vi "vis_com_RW.vi"(6 "SerialSetting":T1={"Baud Rate"=115200, "Data Bits"=8, "Parity"=0, "Stop Bits"=10} {"Stop Bits" items=["1.0"=10, "1.5"=15, "2.0"=20]; "Parity" items=["None", "Odd", "Even", "Mark", "Space"]}, 7 "Funciton":T2, 8 "error in (no error)":errorcluster, 9 "TermChar":string="\n", 10 "CMD String":string, 11 "VISA resource in":refnum<visa-resource-name>) -> (0 "error out":errorcluster, 2 "Result":string, 3 "VISA resource out":refnum<visa-resource-name>)   [LabVIEW 2020, in "GPP.lvlib"]
uses:
  GPP.lvlib
  VISA_COMMON.ctl
  Global.vi
panel:
  out "trimmed string":string
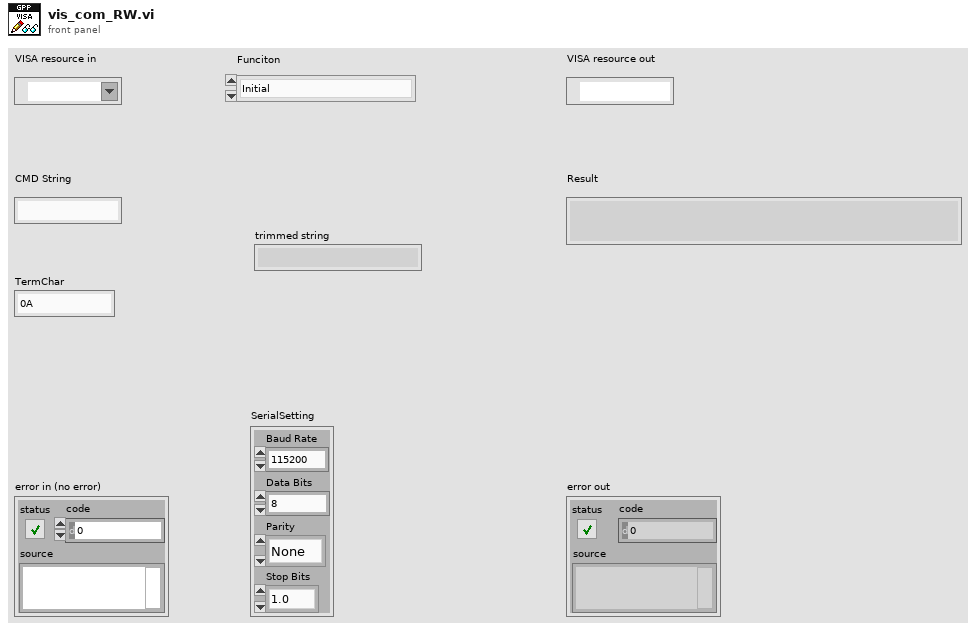
[diagram p1: front panel]
types:
  T1 = cluster{"Baud Rate":u32, "Data Bits":u16, "Parity":u16, "Stop Bits":u16}
  T2 = typedef "GPP.lvlib/VISA_COMMON.ctl" = enum16{"Initial", "Write CMD", "Read Result", "Read History", "Close"}
  T3 = enum16{"open", "replace", "create", "open or create", "replace or create", "replace or create with confirmation"}
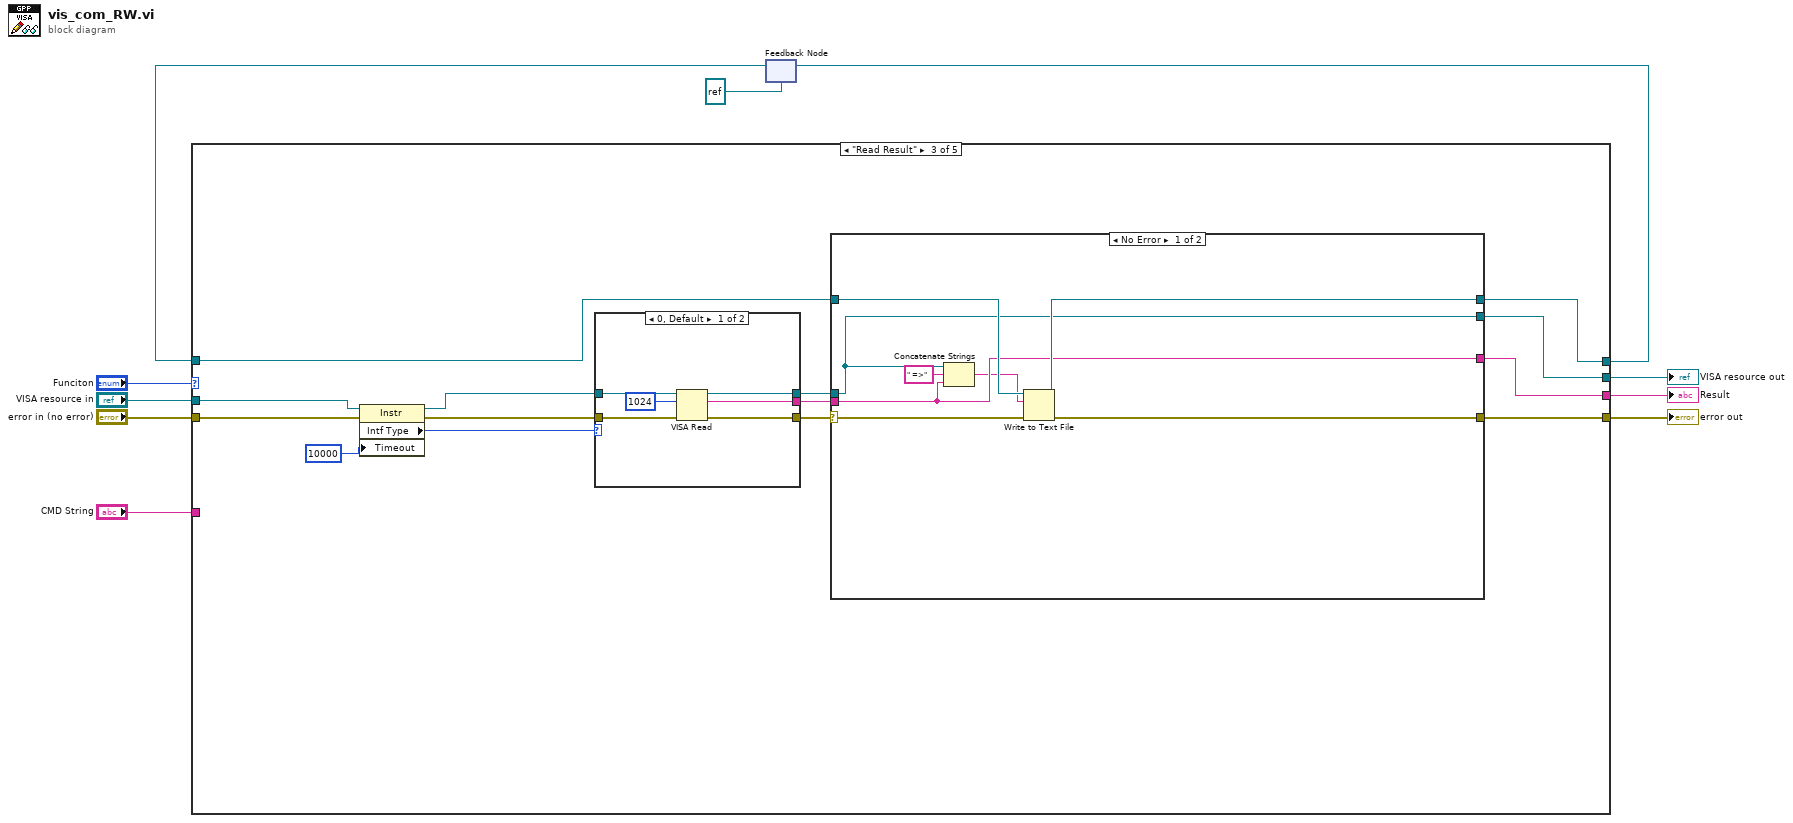
[diagram p0: block diagram]
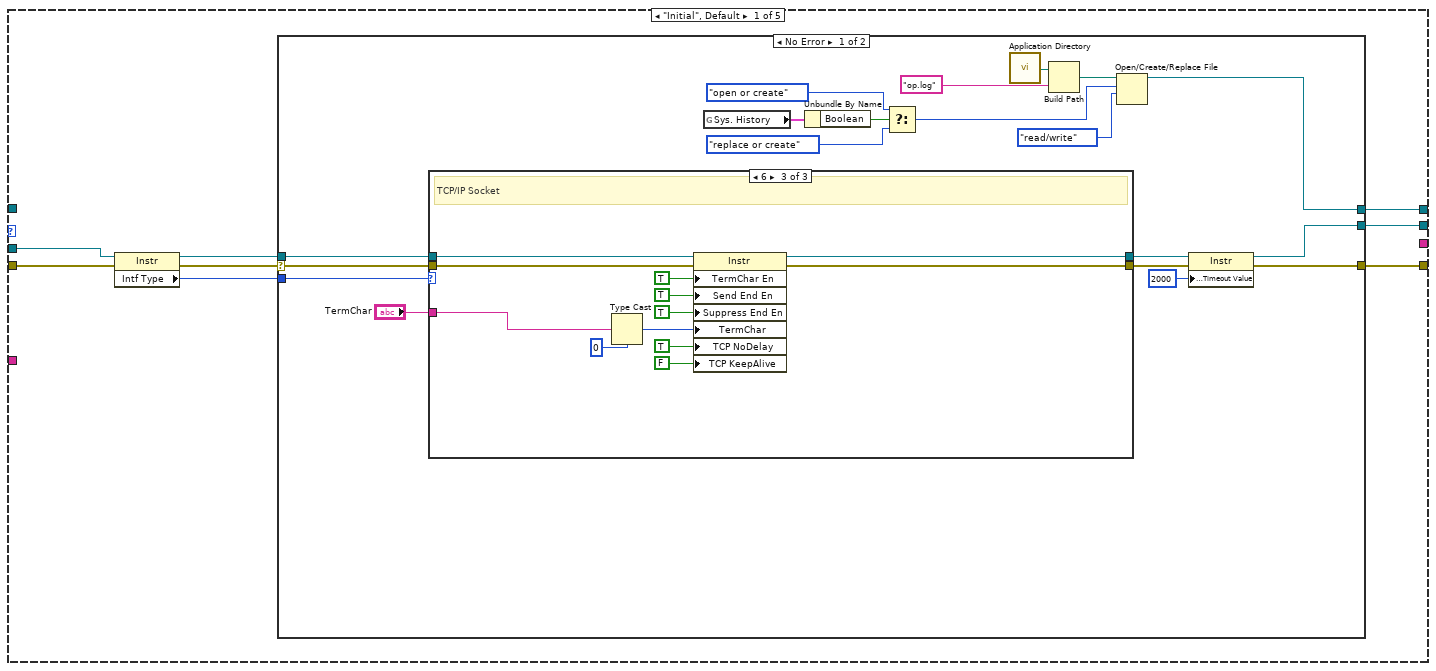
[diagram p2: hidden frame]
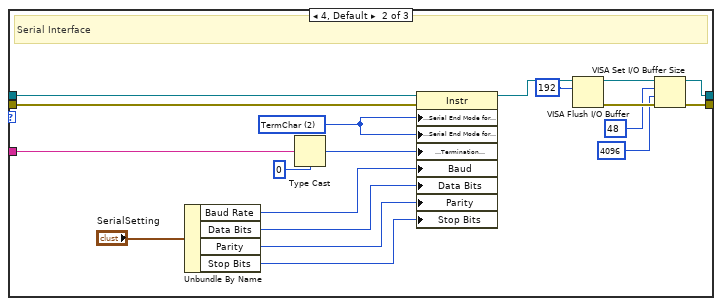
[diagram p4: hidden frame]
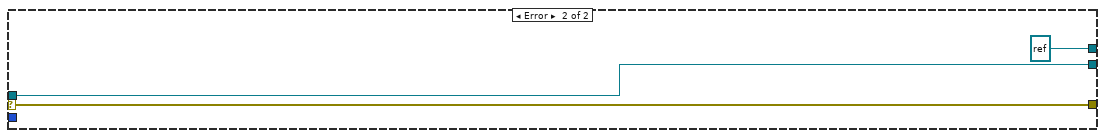
[diagram p5: hidden frame]
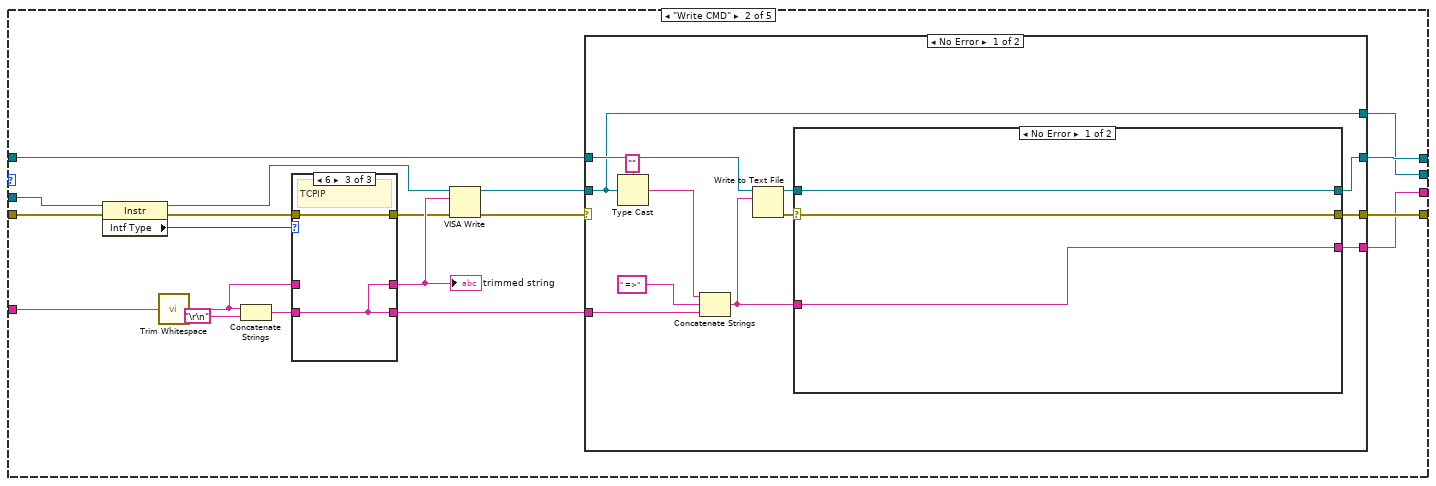
[diagram p6: hidden frame]
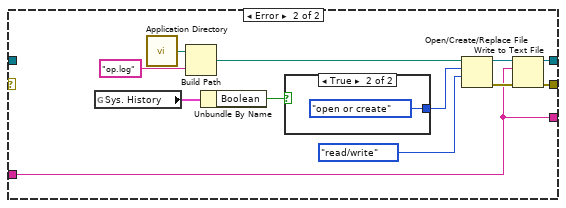
[diagram p9: hidden frame]
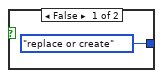
[diagram p10: hidden frame]
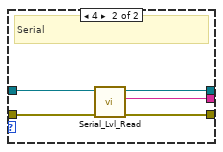
[diagram p12: hidden frame]
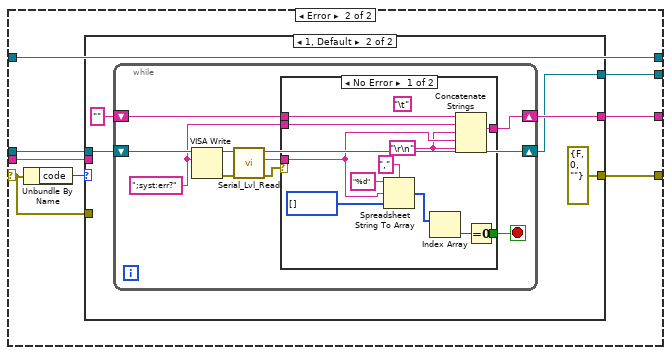
[diagram p13: hidden frame]
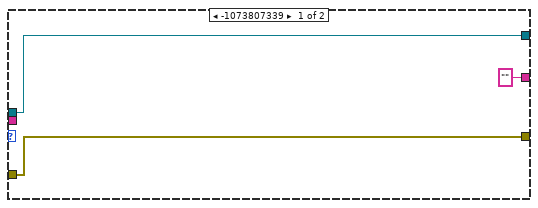
[diagram p14: hidden frame]
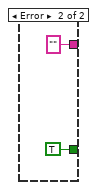
[diagram p15: hidden frame]
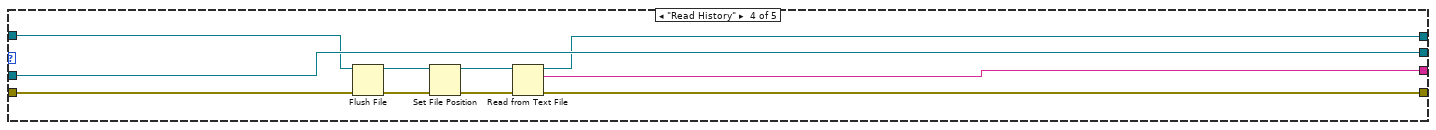
[diagram p16: hidden frame]
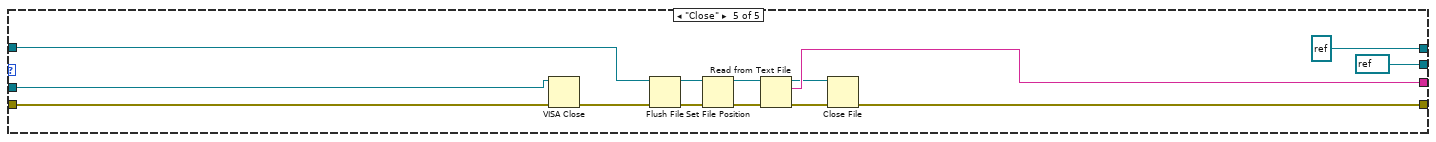
[diagram p17: hidden frame]
diagram:
  n1 = feedback #1(refnum<file> refnum ("refnum out")) -> (w4:refnum<file>)
  n2 = case shown="\"Read Result\"" "Funciton" {
    tunnel: "VISA resource in" -> [w17 w85 w145 w211 w227]
    tunnel: "CMD String" -> [_ w83 _ _ _]
    tunnel: "error in (no error)" -> [w13 w84 w134 w204 w226]
    tunnel: [w12 w91 w143 w212 w221] -> w7
    tunnel: [_ w88 w142 w213 w225] -> w6
    tunnel: [w18 w90 w139 w205 refnum<file> refnum ("refnum out")] -> w3
    tunnel: w4 -> [_ w92 w141 w210 w217]
    tunnel: [w14 w86 w135 w211 refnum<visa-resource-name> refnum ("VISA resource out")] -> w1
    frame "Initial", Default {
      n3 = property class="Instr"(reference=w17, error in=w13) -> (reference out=w15:refnum<visa-resource-name>, error out=w11:errorcluster, "Intf Type"=w16:u16)
      n4 = case shown="No Error" w11 {
        selector: w11 -> [w22 w72]
        tunnel: [w33 refnum<file> refnum ("refnum out")] -> w18
        tunnel: w16 -> [w24 _]
        tunnel: w15 -> [w23 w73]
        tunnel: [w31 w73] -> w14
        tunnel: [w30 w72] -> w12
        frame No Error {
          n5 = case shown="6" w24 {
            tunnel: [w38 w55 w68] -> w21
            tunnel: [w39 w53 w67] -> w20
            tunnel: w23 -> [w38 w57 w70]
            tunnel: w22 -> [w39 w58 w69]
            tunnel: "TermChar" -> [_ w46 w59]
            frame 1 {
              # "GPIB and USB Interface"
            }
            frame 4, Default {
              w47 = u16 2 items=["None", "LastBit", "TermChar"] ("Serial Settings:Serial End Mode for Reads")
              # "Serial Interface"
              n6 = Unbundle By Name("SerialSetting") -> ("Baud Rate"=w44:u32, "Data Bits"=w43:u16, "Parity"=w42:u16, "Stop Bits"=w41:u16)
              n7 = Type Cast(type=u8 0, x=w46) -> (*(type *) &x=w40:u8)
              n8 = property class="Instr"(reference=w57, error in=w58, "Serial Settings:Serial End Mode for Reads"=w47, "Serial Settings:Serial End Mode for Writes"=w47, "Message Based Settings:Termination Character"=w40, "Baud"=w44, "Data Bits"=w43, "Parity"=w42, "Stop Bits"=w41) -> (reference out=w52:refnum<visa-resource-name>)  [unwired: 1 out]
              n9 = VISA Flush I/O Buffer(VISA resource name=w52, mask (16)=u16 192) -> (VISA resource name out=w56:refnum<visa-resource-name>, error out=w54:errorcluster)  [unwired: 1 in]
              n10 = VISA Set I/O Buffer Size(VISA resource name=w56, mask (16)=u16 48, size (4096)=u32 4096 ("size (0)"), error in (no error)=w54) -> (VISA resource name out=w55:refnum<visa-resource-name>, error out=w53:errorcluster)
            }
            frame 6 {
              # "TCP/IP Socket"
              n11 = Type Cast(type=u8 0, x=w59) -> (*(type *) &x=w65:u8)
              n12 = property class="Instr"(reference=w70, error in=w69, "TermChar En"=TRUE ("Message Based Settings:Termination Character Enable"), "Send End En"=TRUE ("Message Based Settings:Send End Enable"), "Suppress End En"=TRUE ("Message Based Settings:Suppress End Enable"), "TermChar"=w65, "TCP NoDelay"=TRUE ("TCP/IP Settings:No Packet Delay"), "TCP KeepAlive"=FALSE ("TCP/IP Settings:Keep-Alive Packets")) -> (reference out=w68:refnum<visa-resource-name>, error out=w67:errorcluster)
            }
          }
          n13 = global read "Global.vi" "Sys. History"() -> (w29:cluster{"Boolean":bool})
          n14 = Unbundle By Name(w29) -> ("Boolean"=w28:bool)
          n15 = Select(t=T3."open or create", s=w28, f=T3."replace or create" ("operation (0:open)")) -> (s? t:f=w27:T3)
          n16 = call <vilib>:"Application Directory.vi"() -> ("Application Directory"=w36:path)
          n17 = Build Path(base path=w36, name or relative path="op.log") -> (appended path=w37:path)
          n18 = Open/Create/Replace File(file path (use dialog)=w37, operation (0:open)=w27, access (0:read/write)=enum16{"read/write", "read-only", "write-only"}."read/write") -> (refnum out=w33:refnum<file>)  [unwired: 3 in, 2 out]
          n19 = property class="Instr"(reference=w21, error in=w20, "General Settings:Timeout Value"=u32 2000) -> (reference out=w31:refnum<visa-resource-name>, error out=w30:errorcluster)
        }
        frame Error {
        }
      }
    }
    frame "Write CMD" {
      n20 = property class="Instr"(reference=w85, error in=w84) -> (reference out=w75:refnum<visa-resource-name>, error out=w77:errorcluster, "Intf Type"=w74:u16)
      n21 = call <vilib>:"Trim Whitespace.vi"("string"=w83) -> ("trimmed string"=w79:string)  [unwired: 1 in]
      n22 = Concatenate Strings(w79, "\r\n") -> (w78:string)
      n23 = case shown="6" w74 {
        tunnel: w79 -> [w93 w97 _]
        tunnel: [w93 w96 w99] -> w81
        tunnel: [w93 w97 w99] -> w82
        tunnel: w78 -> [_ w96 w99]
        tunnel: w77 -> [w94 w95 w98]
        tunnel: [w94 w95 w98] -> w76
        frame 0, Default {
        }
        frame 4 {
          # "Serial"
        }
        frame 6 {
          # "TCPIP"
        }
      }
      "trimmed string" <- w82
      n24 = VISA Write(VISA resource name=w75, write buffer=w82, error in (no error)=w76) -> (VISA resource name out=w89:refnum<visa-resource-name>, error out=w87:errorcluster)  [unwired: 1 out]
      n25 = case shown="No Error" w87 {
        selector: w87 -> [_ w130]
        tunnel: w92 -> [w111 w131]
        tunnel: [w109 w130] -> w91
        tunnel: [w108 w131] -> w90
        tunnel: w81 -> [w106 _]
        tunnel: w89 -> [w101 w129]
        tunnel: [w105 _] -> w88
        tunnel: [w101 w129] -> w86
        frame No Error {
          n26 = Type Cast(type="" ("string"), x=w101) -> (*(type *) &x=w100:string)
          n27 = Concatenate Strings(w100, " =>" ("string"), w106) -> (w103:string)
          n28 = Write to Text File(file (use dialog)=w111, text=w103) -> (refnum out=w107:refnum<file>, error out=w110:errorcluster)  [unwired: 2 in, 1 out]
          n29 = case shown="No Error" w110 {
            selector: w110 -> [w114 _]
            tunnel: [w114 w122] -> w109
            tunnel: [w113 w120] -> w108
            tunnel: w107 -> [w113 _]
            tunnel: [w112 w115] -> w105
            tunnel: w103 -> [w112 w115]
            frame No Error {
            }
            frame Error {
              n30 = global read "Global.vi" "Sys. History"() -> (w118:cluster{"Boolean":bool})
              n31 = call <vilib>:"Application Directory.vi"() -> ("Application Directory"=w119:path)
              n32 = Build Path(base path=w119, name or relative path="op.log") -> (appended path=w126:path)
              n33 = Unbundle By Name(w118) -> ("Boolean"=w117:bool)
              n34 = case shown="True" w117 {
                tunnel: [T3."replace or create" ("operation (0:open)") T3."open or create" ("operation (0:open)")] -> w116
                frame False {
                }
                frame True {
                }
              }
              n35 = Open/Create/Replace File(file path (use dialog)=w126, operation (0:open)=w116, access (0:read/write)=enum16{"read/write", "read-only", "write-only"}."read/write") -> (refnum out=w121:refnum<file>, error out=w123:errorcluster)  [unwired: 3 in, 1 out]
              n36 = Write to Text File(file (use dialog)=w121, text=w115, error in=w123) -> (refnum out=w120:refnum<file>, error out=w122:errorcluster)  [unwired: 1 in, 1 out]
            }
          }
        }
        frame Error {
        }
      }
    }
    frame "Read Result" {
      n37 = property class="Instr"(reference=w145, error in=w134, "Timeout"=10000) -> (reference out=w137:refnum<visa-resource-name>, error out=w133:errorcluster, "Intf Type"=w136:u16)
      n38 = case shown="0, Default" w136 {
        tunnel: w137 -> [w151 w156]
        tunnel: w133 -> [w150 w155]
        tunnel: [w149 w152] -> w144
        tunnel: [w147 w153] -> w140
        tunnel: [w146 w154] -> w138
        frame 0, Default {
          n39 = VISA Read(VISA resource name=w151, byte count=u32 1024, error in (no error)=w150) -> (VISA resource name out=w146:refnum<visa-resource-name>, read buffer=w147:string, error out=w149:errorcluster)  [unwired: 1 out]
        }
        frame 4 {
          # "Serial"
          n40 = call "Serial_Lvl_Read.vi"("error in (no error)"=w155, "VISA Refnum in"=w156) -> ("error out"=w152:errorcluster, "read buffer"=w153:string, "VISA Refnum out"=w154:refnum<visa-resource-name>)  [unwired: 6 in, 1 out]
        }
      }
      n41 = case shown="No Error" w144 {
        selector: w144 -> [w163 w167]
        tunnel: [w158 w166] -> w143
        tunnel: w140 -> [w161 w165]
        tunnel: [w161 w171] -> w142
        tunnel: w141 -> [w164 w172]
        tunnel: [w162 w172] -> w139
        tunnel: w138 -> [w157 w170]
        tunnel: [w157 w169] -> w135
        frame No Error {
          n42 = Concatenate Strings(w157, " =>" ("string"), w161) -> (w160:string)
          n43 = Write to Text File(file (use dialog)=w164, text=w160, error in=w163) -> (refnum out=w162:refnum<file>, error out=w158:errorcluster)  [unwired: 1 in, 1 out]
        }
        frame Error {
          n44 = Unbundle By Name(w167) -> ("code"=w168:i32)
          n45 = case shown="1, Default" w168 {
            tunnel: ["" w180] -> w171
            tunnel: w170 -> [w175 w178]
            tunnel: [w175 w177] -> w169
            tunnel: w167 -> [w173 _]
            tunnel: [w173 errorcluster {"status"=FALSE, "code"=0, "source"=""} ("error IO")] -> w166
            tunnel: w165 -> [_ _]
            frame -1073807339 {
            }
            frame 1, Default {
              n46 = while {
                shift-right: [w187] -> w180
                shift-left: "" -> [w189]
                shift-right: [w184] -> w177
                shift-left: w178 -> [w190]
                stop <- w186 stop-if-true
                w188 = ";syst:err?" ("name or relative path")
                n47 = VISA Write(VISA resource name=w190, write buffer=w188) -> (VISA resource name out=w185:refnum<visa-resource-name>, error out=w182:errorcluster)  [unwired: 1 in, 1 out]
                n48 = call "Serial_Lvl_Read.vi"("error in (no error)"=w182, "VISA Refnum in"=w185) -> ("error out"=w181:errorcluster, "read buffer"=w183:string, "VISA Refnum out"=w184:refnum<visa-resource-name>)  [unwired: 6 in, 1 out]
                n49 = case shown="No Error" w181 {
                  tunnel: w189 -> [w201 _]
                  tunnel: w188 -> [w200 _]
                  tunnel: [w199 ""] -> w187
                  tunnel: [w198 TRUE] -> w186
                  tunnel: w183 -> [w192 _]
                  frame No Error {
                    (unwired) "\t"
                    w191 = "\r\n"
                    n50 = Spreadsheet String To Array(delimiter (Tab)=",", format string="%d", spreadsheet string=w192, array type (2D Dbl)=i32[] []) -> (array=w194:i32[])
                    n51 = Index Array(array=w194) -> (element=w193:i32)  [unwired: 1 in]
                    n52 = Concatenate Strings(w201, w200, w191, w192, w191) -> (w199:string)
                    n53 = Equal To 0?(x=w193) -> (x = 0?=w198:bool)
                  }
                  frame Error {
                  }
                }
              }
            }
          }
        }
      }
    }
    frame "Read History" {
      n54 = Flush File(refnum=w210, error in=w204) -> (refnum out=w208:refnum<file>, error out=w209:errorcluster)
      n55 = Set File Position(refnum=w208, error in=w209) -> (refnum out=w207:refnum<file>, error out=w206:errorcluster)  [unwired: 2 in]
      n56 = Read from Text File(file (use dialog)=w207, error in=w206) -> (refnum out=w205:refnum<file>, text=w213:string, error out=w212:errorcluster)  [unwired: 2 in, 1 out]
    }
    frame "Close" {
      n57 = VISA Close(VISA resource name=w227, error in (no error)=w226) -> (error out=w218:errorcluster)
      n58 = Flush File(refnum=w217, error in=w218) -> (refnum out=w216:refnum<file>, error out=w219:errorcluster)
      n59 = Set File Position(refnum=w216, error in=w219) -> (refnum out=w215:refnum<file>, error out=w214:errorcluster)  [unwired: 2 in]
      n60 = Read from Text File(file (use dialog)=w215, error in=w214) -> (refnum out=w224:refnum<file>, text=w225:string, error out=w222:errorcluster)  [unwired: 2 in, 1 out]
      n61 = Close File(refnum=w224, error in=w222) -> (error out=w221:errorcluster)  [unwired: 1 out]
    }
  }
  "error out" <- w7
  "Result" <- w6
  "VISA resource out" <- w1
  n62 = feedback-in #1(w3) -> ()
